vi "Launch Detail View.vi"(8 "error in (no error)":errorcluster, 11 "Sensor in":refnum<class "Sensor.lvclass">) -> (0 "error out":errorcluster, 3 "Sensor out":refnum<class "Sensor.lvclass">)   [LabVIEW 2012, in "Sensor Definition.lvlib" / "Sensor.lvclass"]
uses:
  Sensor.lvclass
  <vilib>/ActorFramework/Actor/Actor.lvclass
  Win8uiFramework/MainPane Slide Msg.lvclass
  Win8uiFramework/Slide Direction.ctl
  Win8uiFramework/Win8uiFramework.lvlib
  HostType.ctl
  Sensor Definition.lvlib
  SensorViewDetailed.lvclass
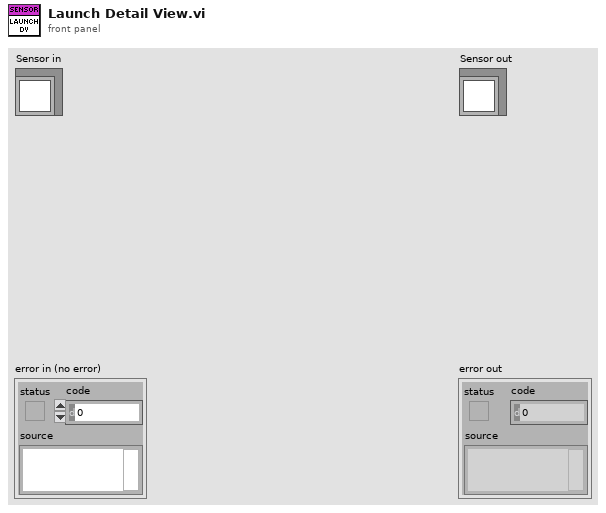
[diagram p1: front panel]
types:
  T1 = typedef "Sensor Definition.lvlib/HostType.ctl" = enum16{"Standalone", "Grid", "MainPane"}
  T2 = typedef "Win8uiFramework.lvlib/Slide Direction.ctl" = enum16{"Forwards", "Back"}
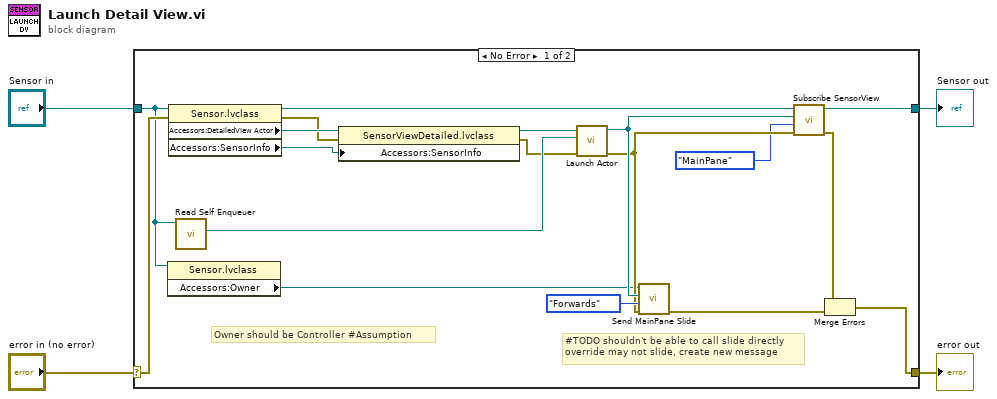
[diagram p0: block diagram]
diagram:
  n1 = case shown="No Error" "error in (no error)" {
    selector: "error in (no error)" -> [w13 w24]
    tunnel: [w12 w24] -> w3
    tunnel: [w21 w23] -> w1
    tunnel: "Sensor in" -> [w11 w23]
    frame No Error {
      # "#TODO shouldn't be able to call slide directly\noverride may not slide, create new message"
      # "Owner should be Controller #Assumption"
      n2 = property class="Sensor.lvclass"(reference=w11) -> ("Accessors:Owner"=w10:refnum<class "Message Enqueuer.lvclass">)  [unwired: 1 in, 2 out]
      n3 = property class="Sensor.lvclass"(reference=w11, error in=w13) -> (reference out=w22:refnum<class "Sensor.lvclass">, error out=w7:errorcluster, "Accessors:DetailedView Actor"=w20:refnum<class "SensorViewDetailed.lvclass">, "Accessors:SensorInfo"=w5:refnum<class "SensorInfo.lvclass">)
      n4 = call <vilib>:"Read Self Enqueuer.vi"("Actor"=w11) -> ("Self Enqueuer"=w19:refnum<class "Message Enqueuer.lvclass">)  [unwired: 10 in]
      n5 = property class="SensorViewDetailed.lvclass"(reference=w20, error in=w7, "Accessors:SensorInfo"=w5) -> (reference out=w8:refnum<class "SensorViewDetailed.lvclass">, error out=w6:errorcluster)
      n6 = call <vilib>:"Launch Actor.vi"("error in (no error)"=w6, "Actor-to-Caller Enqueuer"=w19, "Actor"=w8) -> ("error out"=w14:errorcluster, "Caller-To-Actor Enqueuer"=w17:refnum<class "Message Enqueuer.lvclass">)  [unwired: 7 in]
      n7 = call "Send MainPane Slide.vi"("error in (no error)"=w14, "Slide Direction"=Slide_Direction."Forwards", "Enqueuer"=w17, "Message Enqueuer"=w10) -> ("error out"=w16:errorcluster)  [unwired: 6 in, 1 out]
      n8 = call "Subscribe SensorView.vi"("error in (no error)"=w14, "HostType"=HostType."MainPane", "SensorView Enqueuer"=w17, "Sensor in"=w22) -> ("error out"=w15:errorcluster, "Sensor out"=w21:refnum<class "Sensor.lvclass">)  [unwired: 6 in]
      n9 = Merge Errors(w15, w16) -> (w12:errorcluster)
    }
    frame Error {
    }
  }
  "error out" <- w3
  "Sensor out" <- w1
